vi "Set Set Point-moose.vi"(3 "COM Port IN":refnum<visa-resource-name>="COM12", 8 "Numerical\nSet Value":dbl format="%.2f", 9 "error in\n(no error)":errorcluster) -> (0 "COM Port OUT":refnum<visa-resource-name>="COM12", 1 "Numeric\nReading Value":dbl format="%.2f", 5 "Reading String\nwith Descriptor":string, 6 "error out":errorcluster)   [LabVIEW 2010]
doc: "This VI will independently set the internal Neslab device Set Point."
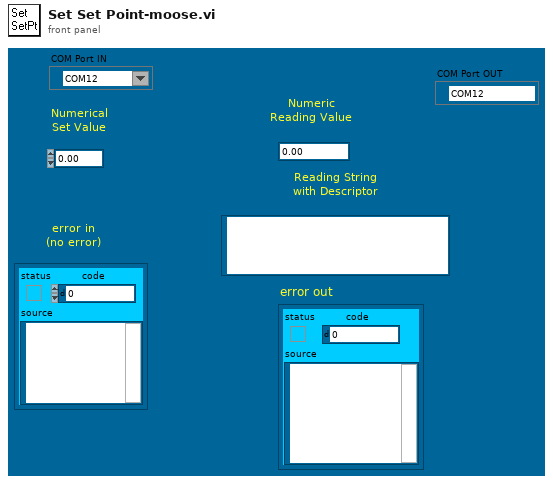
[diagram p1: front panel]
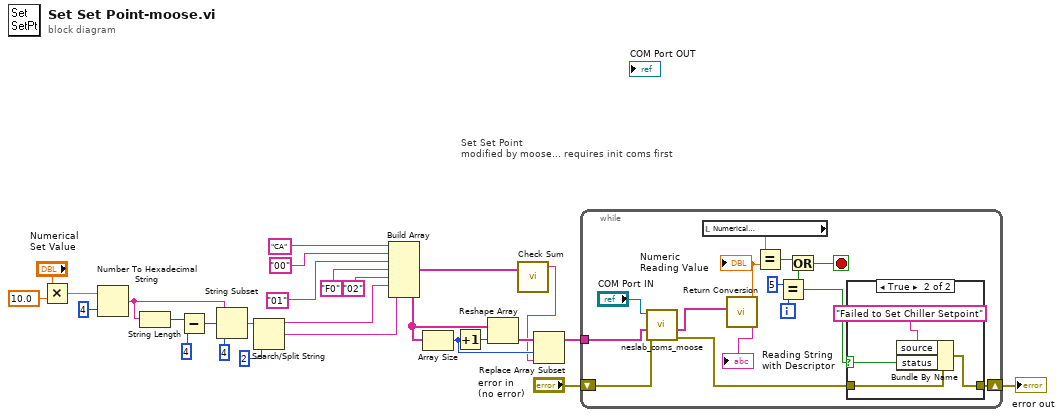
[diagram p0: block diagram]
diagram:
  # "Set Set Point\nmodified by moose... requires init coms first"
  n1 = Multiply(x="Numerical\nSet Value", y=10.0 ("f")) -> (x*y=w2:dbl)
  n2 = Number To Hexadecimal String(1:i16 4 ("width (-)"), 2:w2) -> (0:w14:string)
  n3 = String Length(string=w14) -> (length=w17:i32)
  n4 = Subtract(x=w17, y=4) -> (x-y=w16:i32)
  n5 = String Subset(string=w14, offset (0)=w16, length (rest)=4 ("length (rest)")) -> (substring=w10:string)
  n6 = Search/Split String(string=w10, offset (0)=2) -> (substring before match=w12:string, match + rest of string=w22:string)  [unwired: 1 in, 1 out]
  n7 = Build Array("CA", "00", "01", "F0", "02", w12, w22) -> (w4:string[])
  n8 = Array Size(array=w4) -> (size(s)=w19:i32)
  n9 = Increment(x=w19) -> (x+1=w20:i32)
  n10 = Reshape Array(w4, w20) -> (w23:string[])
  n11 = call "Check Sum.VI"("Input String"=w4) -> ("Checksum"=w1:string)  [unwired: 1 in, 2 out]
  n12 = Replace Array Subset(array=w23, new element=w1, index=w19) -> (w21:string[])
  n13 = while {
    tunnel: w21 -> [w31]
    shift-right: [w32] -> w5
    shift-left: "error in\n(no error)" -> [w30]
    i -> [w37]
    stop <- w33 stop-if-true
    n14 = call "neslab_coms_moose.vi"("error in"=w30, "byte array\n(in)"=w31, "COM Port IN"="COM Port IN") -> ("error out 2"=w28:errorcluster, "byte array\n(out)"=w27:string[])  [unwired: 3 in, 2 out]
    n15 = local read "Numerical\nSet Value"() -> (w39:dbl)
    n16 = call "Return Conversion.VI"("Input Array"=w27) -> ("Numeric\nReading\nValue"=w38:dbl, "Reading String\nwith Descriptor"=→"Reading String\nwith Descriptor":string)  [unwired: 7 in]
    "Numeric\nReading Value" <- w38
    n17 = Equal?(x=w39, y=w38) -> (x = y?=w35:bool)
    n18 = Equal?(x=5, y=w37) -> (x = y?=w34:bool)
    n19 = Or(x=w35, y=w34) -> (x .or. y?=w33:bool)
    n20 = case shown="True" w34 {
      selector: w34 -> [_ w44]
      tunnel: w28 -> [w41 w45]
      tunnel: [w41 w43] -> w32
      frame False {
      }
      frame True {
        n21 = Bundle By Name(cluster=w45, "source"="Failed to Set Chiller Setpoint", "status"=w44) -> (w43:errorcluster)
      }
    }
  }
  "error out" <- w5
